vi "System Definition To Ports.vi"(8 "error in":errorcluster, 11 "custom device ref":T1 format="%.0x") -> (0 "error out":errorcluster, 2 "ports":T2[](array[typedef]), 3 "custom device ref out":T1 format="%.0x")   [LabVIEW 2020, in "AIM ARINC 429 Scripting.lvlib"]
uses:
  AIM ARINC 429 Scripting.lvlib
  <vilib>/NI VeriStand/Custom Device API/Custom Device Item Ref.ctl
  Shared/VS Channels Definition for All Labels on Hardware Channel.ctl
  Shared/Direction.ctl
  Shared/VS Channels Definition for Label.ctl
  Shared/VS Channel Definition for Parameter.ctl
  Shared/Parameter Definition.ctl
  <vilib>/NI/NI VeriStand Encoding and Decoding/Encoding.ctl
  Shared/Transfer Type.ctl
  <vilib>/NI/NI VeriStand Encoding and Decoding/Encoding and Decoding.lvlib
  ARINC 429/ARINC 429 Scripting.lvlib
  <vilib>/NI VeriStand/Custom Device API/Custom Device API.lvlib
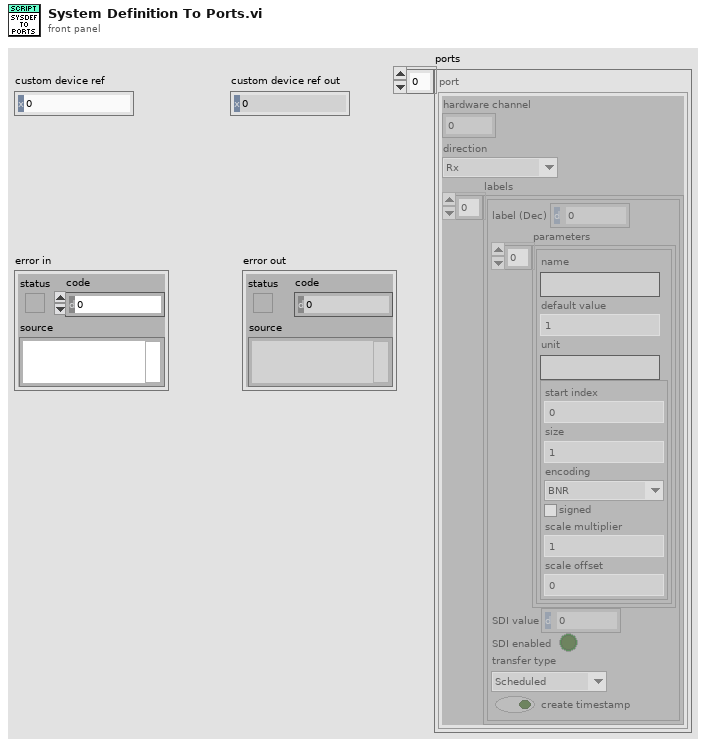
[diagram p1: front panel]
types:
  T1 = typedef "Custom Device API.lvlib/Custom Device Item Ref.ctl" = u64
  T2 = typedef "VS Channels Definition for All Labels on Hardware Channel.ctl" = cluster{"hardware channel":i32, "direction":T3, "labels":T4[]}
  T3 = typedef "Direction.ctl" = enum16{"Rx", "Tx"}
  T4 = typedef "VS Channels Definition for Label.ctl" = cluster{"label (Dec)":u32, "parameters":T5[], "SDI value":u8, "SDI enabled":bool, "transfer type":T8, "create timestamp":bool}
  T5 = typedef "VS Channel Definition for Parameter.ctl" = cluster{"name":string, "default value":dbl, "unit":string, "Parameter":T6}
  T6 = typedef "Parameter Definition.ctl" = cluster{"start index":i32, "size":i32, "encoding":T7, "signed":bool, "scale multiplier":dbl, "scale offset":dbl}
  T7 = typedef "Encoding and Decoding.lvlib/Encoding.ctl" = enum16{"BNR", "BCD", "Discrete"}
  T8 = typedef "Transfer Type.ctl" = enum16{"Scheduled", "Acyclic", "Block", "Strobe"}
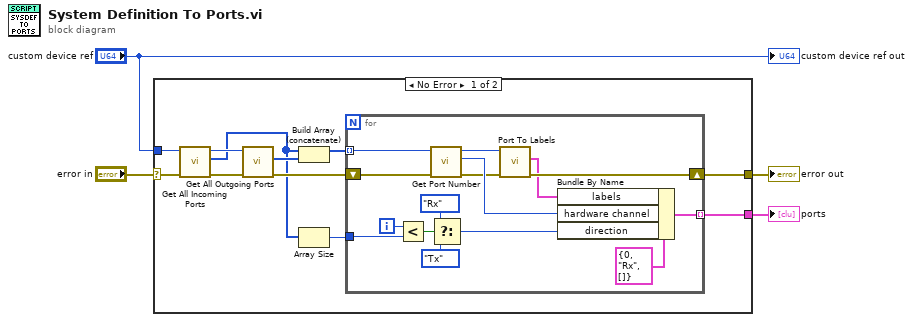
[diagram p0: block diagram]
diagram:
  n1 = case shown="No Error" "error in" {
    selector: "error in" -> [w14 w31]
    tunnel: "custom device ref" -> [w15 _]
    tunnel: [w7 w31] -> w4
    tunnel: [w8 _] -> w1
    frame No Error {
      n2 = call "Get All Incoming Ports.vi"("error in"=w14, "Ballard ARINC 429 custom device in"=w15) -> ("error out"=w13:errorcluster, "incoming ports"=w5:T1[], "Ballard ARINC 429 custom device out"=w11:T1)  [unwired: 7 in]
      n3 = call "Get All Outgoing Ports.vi"("error in"=w13, "Ballard ARINC 429 custom device in"=w11) -> ("error out"=w9:errorcluster, "outgoing ports"=w12:T1[])  [unwired: 7 in, 1 out]
      n4 = Build Array (concatenate)(w5, w12) -> (w10:T1[])
      n5 = Array Size(array=w5) -> (size(s)=w6:i32)
      n6 = for {
        tunnel: w10 -> [w29] mode=indexing
        shift-right: [w18] -> w7
        shift-left: w9 -> [w30]
        tunnel: [w26] -> w8 mode=indexing
        tunnel: w6 -> [w21]
        i -> [w22]
        n7 = Less?(x=w22, y=w21) -> (x < y?=w23:bool)
        n8 = call "Get Port Number.vi"("error in"=w30, "port ref in"=w29) -> ("error out"=w20:errorcluster, "port number"=w27:u16, "port ref out"=w19:T1)  [unwired: 6 in, 1 out]
        n9 = Select(t=Direction."Rx" ("direction"), s=w23, f=Direction."Tx" ("direction")) -> (s? t:f=w16:T3)
        n10 = call "Port To Labels.vi"("error in"=w20, "port ref"=w19) -> ("error out"=w18:errorcluster, "labels"=w17:T4[])  [unwired: 7 in, 1 out]
        n11 = Bundle By Name(cluster=T2 {"hardware channel"=0, "direction"=enum."Rx", "labels"=[]} ("port"), "labels"=w17, "hardware channel"=w27, "direction"=w16) -> (w26:T2)
      }
    }
    frame Error {
    }
  }
  "error out" <- w4
  "ports" <- w1
  "custom device ref out" <- "custom device ref"
